vi "Find Devices of Specified Type.vi"(8 "error in (no error)":errorcluster, 9 "Measurement Name":string, 10 "Hardware Type":string, 11 "Client Controller in":refnum<class "Client Controller.lvclass">) -> (0 "error out":errorcluster, 3 "Client Controller out":refnum<class "Client Controller.lvclass">)   [LabVIEW 2026, in "Client Controller.lvlib" / "Client Controller.lvclass"]
uses:
  Client Controller.lvclass
  C:/Users/E2013170/Documents/GitHub/Measurement-Utility-Reference/components/MAL-Framework/user.lib/Common Components/Controller/Controller.lvclass
  MAL-Framework/user.lib/Common Components/Controller/Messages/Respond with Devices for Measurement Msg/Respond with Devices for Measurement Msg.lvclass
  C:/Program Files/National Instruments/LabVIEW 2026/vi.lib/ActorFramework/Message/Message.lvclass
  MAL-Framework/user.lib/Common Components/Controller/Messages/Respond with Devices for Measurement Msg/Respond with Devices for Measurement Msg.lvclass/Respond with Devices for Measurement Msg.ctl
  Client Controller.lvclass/Client Controller.ctl
  <vilib>/ActorFramework/Message Enqueuer/Message Enqueuer.lvclass
  recovery/packages/ni_lib_linked_network_actor-1.2.0.19-9492AF5A82/File Group 0/vi.lib/NI/Actors/Linked Network Actor/Linked Network Actor Messages/Transmit Network Message Msg/Transmit Network Message Msg.lvclass
  MAL-Framework/user.lib/Common Components/Controller/Controller.lvclass
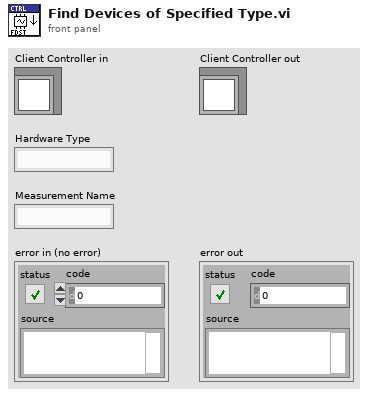
[diagram p1: front panel]
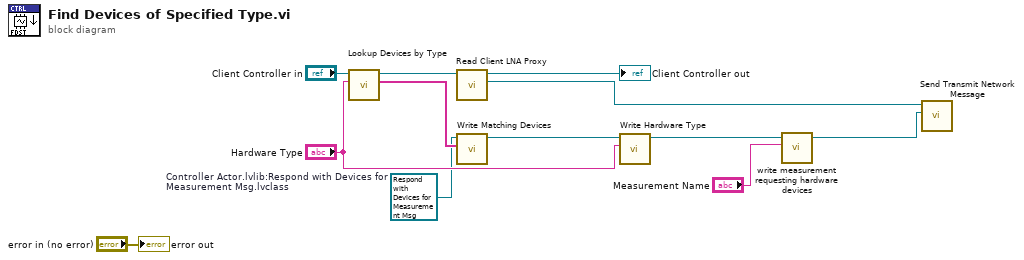
[diagram p0: block diagram]
diagram:
  w5 = refnum<class "Respond with Devices for Measurement Msg.lvclass"> refnum  # Controller Actor.lvlib:Respond with Devices for Measurement Msg.lvclass
  n1 = call "Lookup Devices by Type.vi"("Hardware Type"="Hardware Type", "Controller in"="Client Controller in") -> ("Matching Devices"=w6:string[], "Controller out"=w8:refnum<class "Client Controller.lvclass">)  [unwired: 7 in, 1 out]
  n2 = call "Read Client LNA Proxy.vi"("Client Controller in"=w8) -> ("Actor Framework:Message Enqueuer"=w11:refnum<class "Message Enqueuer.lvclass">, "Client Controller out"=→"Client Controller out":refnum<class "Client Controller.lvclass">)  [unwired: 8 in, 1 out]
  n3 = call "Write Matching Devices.vi"("Matching Devices"=w6, "Respond with Devices for Measurement Msg in"=w5) -> ("Respond with Devices for Measurement Msg out"=w4:refnum<class "Respond with Devices for Measurement Msg.lvclass">)  [unwired: 9 in]
  n4 = call "Write Hardware Type.vi"("Hardware Type"="Hardware Type", "Respond with Devices for Measurement Msg in"=w4) -> ("Respond with Devices for Measurement Msg out"=w3:refnum<class "Respond with Devices for Measurement Msg.lvclass">)  [unwired: 9 in]
  n5 = call "write measurement requesting hardware devices.vi"("Measurement Name"="Measurement Name", "Respond with Devices for Measurement Msg in"=w3) -> ("Respond with Devices for Measurement Msg out"=w2:refnum<class "Respond with Devices for Measurement Msg.lvclass">)  [unwired: 9 in]
  n6 = call "Send Transmit Network Message.vi"("Message"=w2, "Message Enqueuer"=w11) -> ()  [unwired: 8 in, 2 out]
  "error out" <- "error in (no error)"
